vi "Setup Set Cluster Values from JSON String.vi"() -> (0 "error out":errorcluster, 2 "JSON string":string="{\n\t\"Width\":640,\n\t\"Height\":480,\n\t\"Sensor\":\"A700\",\n    \"TriggerMode\":0,\n    \"TriggerSource\":1,\n    \"TriggerActivation\":0,\n    \"TriggerSelector\":0,\n    \"AcquisitionMode\":2,\n    \"OutputImageType\":7,\n    \"AcquisitionFrameRate\":1.0,\n    \"AcquisitionFrameCount\":100,\n    \"Timeout\":20000,\n    \"FocusPos\":58000,\n    \"IncompleteBufferMode\":1,\n    \"IRFormat\":0,\n    \"NUCMode\":0,\n    \"NoiseReduction\":0\n}", 3 "Cluster Refnum out":refnum<vi>)   [LabVIEW 2023]
panel:
  in  "Cluster":T1 {"IRFormat" items=["Option0", "Option1"]}
  # "This VI is for Set Cluster Values from JSON String.lvtest"
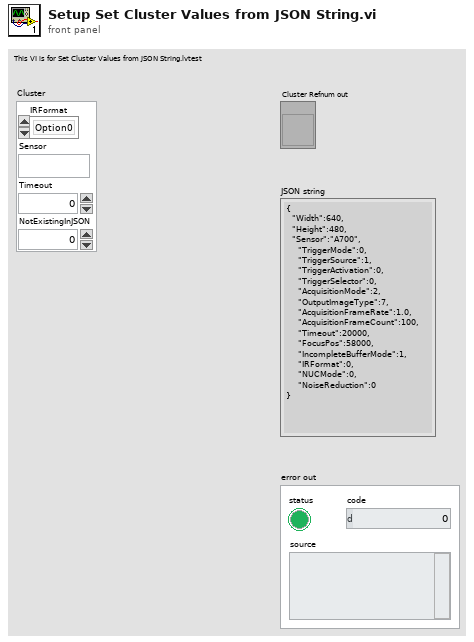
[diagram p1: front panel]
types:
  T1 = cluster{"IRFormat":u16, "Sensor":string, "Timeout":dbl, "NotExistingInJSON":dbl}
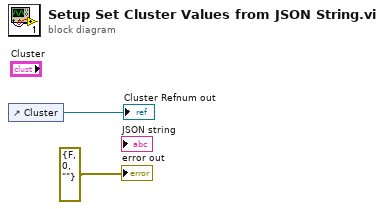
[diagram p0: block diagram]
diagram:
  n1 = control-ref of="Cluster"() -> (→"Cluster Refnum out":refnum<vi>)
  "error out" <- errorcluster {"status"=FALSE, "code"=0, "source"=""} ("error in (no error)")
